vi "ultrasonic align.vi"(8 "error in (no error)":errorcluster, 9 "Enum":enum16{"left", "right"}(ring), 10 "target":dbl format="%#_13g") -> (0 "error out":errorcluster)   [LabVIEW 2019]
uses:
  <vilib>/Platform/TimedLoop/XDataNode/timing_clust.ctl
  <vilib>/Platform/TimedLoop/XDataNode/nitl_modes.ctl
  <vilib>/Platform/TimedLoop/XDataNode/wakeup.ctl
  <vilib>/platform/TimedLoop/XDataNode/XDataNode.xnode
  <vilib>/Platform/TimedLoop/XDataNode/XDNodeRunTimeDep.lvlib
panel:
  in  "stop":bool
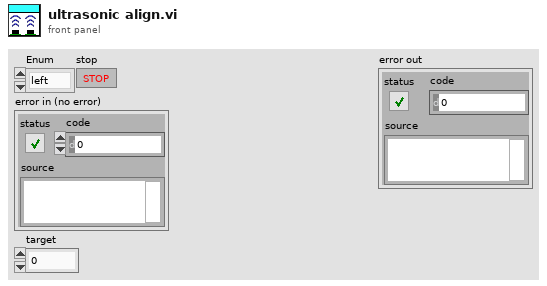
[diagram p1: front panel]
types:
  T1 = typedef "I2C.lvlib/I2C Reference.ctl" = cluster{"myRIO Reference":T2, "I2C Channels Enum":T6, "I2C Configuration":T7}
  T2 = typedef "myRIO Generic Hardware Reference.ctl" = cluster{"myRIO Model":T3, "myRIO Hardware Reference":T4}
  T3 = typedef "Hardware Version Enum.ctl" = enum16{"Unknown", "myRIO-1900", "myRIO-1950", "roboRIO", "NI ELVIS RIO CM", "ELVIS III"}
  T4 = typedef "myRIO v1.0 Reference.ctl" = cluster{"Generic FPGA Reference":T5, "Allow multiple opens":bool}
  T5 = typedef "Generic FPGA Reference.ctl" = refnum<k20>
  T6 = typedef "I2C Channels Enum.ctl" = enum16{"Not Connected", "A/I2C", "B/I2C", "I2C/I2C"}
  T7 = typedef "I2C.lvlib/I2C Configuration.ctl" = cluster{"I2C Transfer Rate":T8}
  T8 = typedef "I2C.lvlib/I2C Transfer Rate.ctl" = enum16{"Standard mode (100 kbps)", "Fast mode (400 kbps)"}
  T9 = typedef "XDNodeRunTimeDep.lvlib/timing_clust.ctl" = cluster{"Expected End [f-1]":u64, "Actual End [f-1]":u64, "Finished Late? [f-1]":bool, "Expected End [i-1]":u64, "Actual End [i-1]":u64, "Finished Late? [i-1]":bool, "Expected Start [i]":u64, "Actual Start [i]":u64, "Expected Start [f]":u64, "Actual Start [f]":u64, "Source Name":string, "Structure Name":string, "Period":i64, "Deadline":i64, "Offset":i64, "Start":i64, "Priority":i32, "Timeout":i32, "Mode":T10, "Wakeup Reason":T11, "Error":errorcluster, "Source Type":string, "Secondary Source Type":string, "Global End Time":u64, "Global Start Time":u64, "Frame Duration":u64, "Iteration Duration":u64, "Assigned CPU":i32, "I/O Scan Engine Mode":u32}
  T10 = typedef "XDNodeRunTimeDep.lvlib/nitl_modes.ctl" = enum32{"No Change", "Process missed periods, maintain original phase", "Discard missed periods, maintain original phase", "Process missed periods, ignore original phase", "Discard missed periods, ignore original phase"}
  T11 = typedef "XDNodeRunTimeDep.lvlib/wakeup.ctl" = enum32{"Normal", "Aborted", "Asynchronous wakeup", "Timing source error", "Timed loop error", "Timeout"}
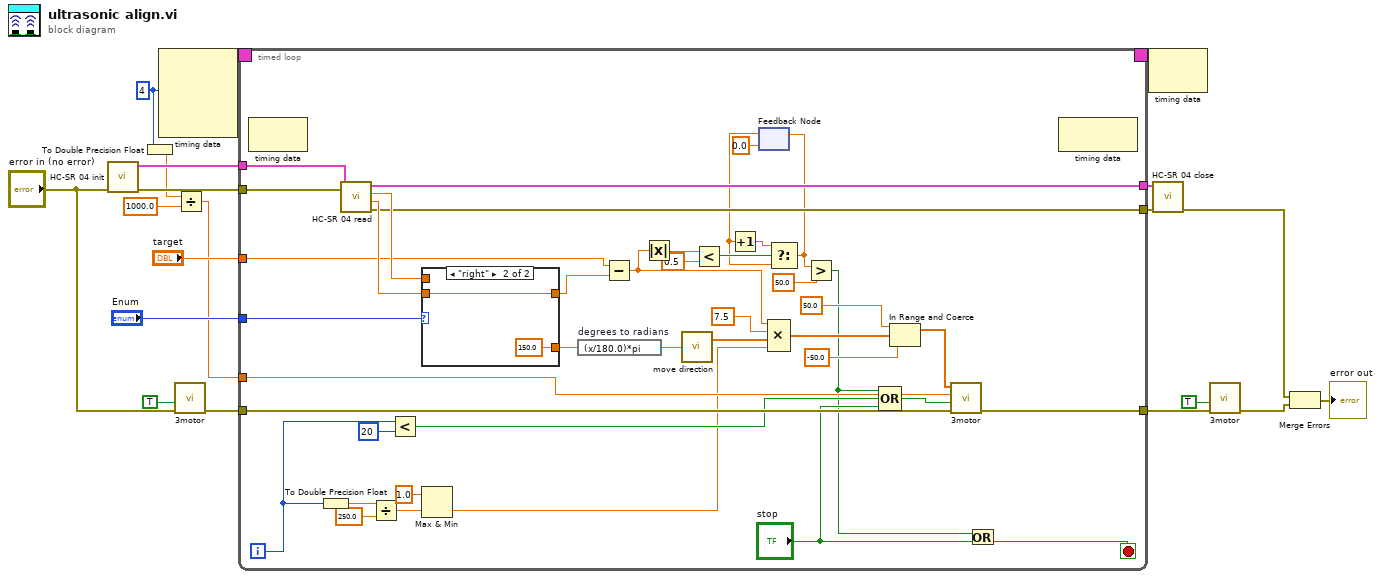
[diagram p0: block diagram]
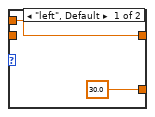
[diagram p2: hidden frame]
diagram:
  w11 = i64 4 ("Period")
  n1 = call "HC-SR 04 init.vi"("error in (no error)"="error in (no error)") -> ("error out"=w16:errorcluster, "I2C Ref Out"=w17:T1)  [unwired: 9 in]
  n2 = To Double Precision Float(number=w11) -> (double precision float=w9:dbl)
  n3 = node-c288(w11) -> (w19:T9)  [unwired: 3 in]
  n4 = call "3motor.vi"("error in (no error)"="error in (no error)", "Reset"=TRUE) -> ("error out"=w12:errorcluster)  [unwired: 9 in]
  n5 = Divide(x=w9, y=1000.0) -> (x/y=w7:dbl)
  n6 = timed-loop {
    timing: w19 -> [_]
    timing-out: [_] -> w18
    tunnel: "Enum" -> [w61]
    tunnel: w17 -> [w60]
    tunnel: w16 -> [w59]
    tunnel: [w56] -> w15
    tunnel: [w55] -> w14
    tunnel: "target" -> [w52]
    tunnel: w12 -> [w45]
    tunnel: w7 -> [w43]
    tunnel: [w42] -> w5
    i -> [w33]
    stop <- w31 stop-if-true
    n7 = node-c288() -> ()  [unwired: 1 in, 1 out]
    n8 = To Double Precision Float(number=w33) -> (double precision float=w37:dbl)
    n9 = call "HC-SR 04 read.vi"("error in (no error)"=w59, "I2C Ref Out in"=w60) -> ("error out"=w55:errorcluster, "Right"=w58:dbl, "Left"=w57:dbl, "I2C Ref Out out"=w56:T1)  [unwired: 5 in, 1 out]
    n10 = Divide(x=w37, y=250.0) -> (x/y=w35:dbl)
    n11 = Less?(x=w33, y=20) -> (x < y?=w38:bool)
    n12 = case shown="\"right\"" w61 {
      tunnel: w58 -> [_ w65]
      tunnel: w57 -> [w63 _]
      tunnel: [w63 w65] -> w51
      tunnel: [30.0 150.0] -> w54
      frame "left", Default {
      }
      frame "right" {
      }
    }
    n13 = Max & Min(x=1.0, y=w35) -> (min(x,y)=w32:dbl)  [unwired: 1 out]
    n14 = expression code="(x/180.0)*pi" "degrees to radians"(w54) -> (w53:dbl)
    n15 = Subtract(x=w52, y=w51) -> (x-y=w30:dbl)
    n16 = Absolute Value(x=w30) -> (abs(x)=w29:dbl)
    n17 = call "move direction.vi"("theta"=w53) -> ("out array"=w50:dbl[])  [unwired: 1 out]
    n18 = Less?(x=w29, y=0.5) -> (x < y?=w27:bool)
    n19 = feedback #1(0.0) -> (w24:dbl)
    n20 = Increment(x=w24) -> (x+1=w26:dbl)
    n21 = Compound Arithmetic op=MULTIPLY(w30, 7.5 ("value"), w50, w32) -> (w46:dbl[])
    n22 = Select(t=w26, s=w27, f=w24) -> (s? t:f=w23:dbl)
    n23 = feedback-in #1(w23) -> ()
    n24 = Greater?(x=w23, y=50.0) -> (0:w21:bool)
    n25 = Compound Arithmetic op=OR(w21, w38, "stop") -> (w40:bool)
    n26 = In Range and Coerce(upper limit=50.0, x=w46, lower limit=-50.0) -> (coerced(x)=w44:dbl[])  [unwired: 1 out]
    n27 = call "3motor.vi"("error in (no error)"=w45, "Reset"=w40, "dt(s)"=w43, "Motor speed"=w44) -> ("error out"=w42:errorcluster)  [unwired: 7 in]
    n28 = Or(x=w21, y="stop") -> (x .or. y?=w31:bool)
    n29 = node-c288() -> ()  [unwired: 1 in, 1 out]
  }
  n30 = node-c288(w18) -> ()  [unwired: 1 out]
  n31 = call "HC-SR 04 close.vi"("error in (no error)"=w14, "I2C Ref Out"=w15) -> ("error out"=w2:errorcluster)  [unwired: 9 in]
  n32 = call "3motor.vi"("error in (no error)"=w5, "Reset"=TRUE) -> ("error out"=w3:errorcluster)  [unwired: 9 in]
  n33 = Merge Errors(w2, w3) -> (→"error out":errorcluster)
